vi "pulsedRead.vi"(0 "osc in":refnum<visa-resource-name>, 1 "connection ID":refnum<k5>, 2 "recCycles":u64=40, 5 "channel":u8, 6 "error in (no error)":errorcluster, 7 "freq (MHz)":dbl=1.367, 9 "cycles":u64=30, 11 "points":u64=80000, 12 "SEQ IN":u32) -> (3 "connection ID out":refnum<k5>, 4 "osc out":refnum<visa-resource-name>, 10 "error out":errorcluster, 13 "voltage":dbl[](array[numeric]), 14 "SEQ OUT":u32, 15 "time":dbl[](array[numeric]))   [LabVIEW 2016]
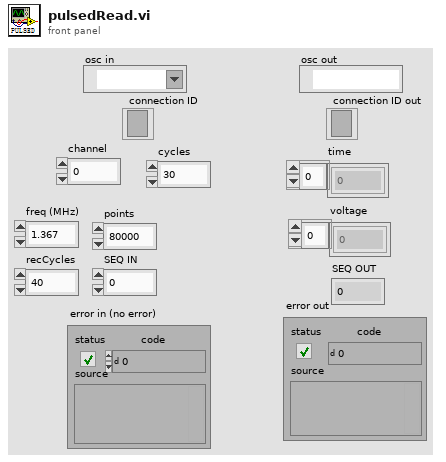
[diagram p1: front panel]
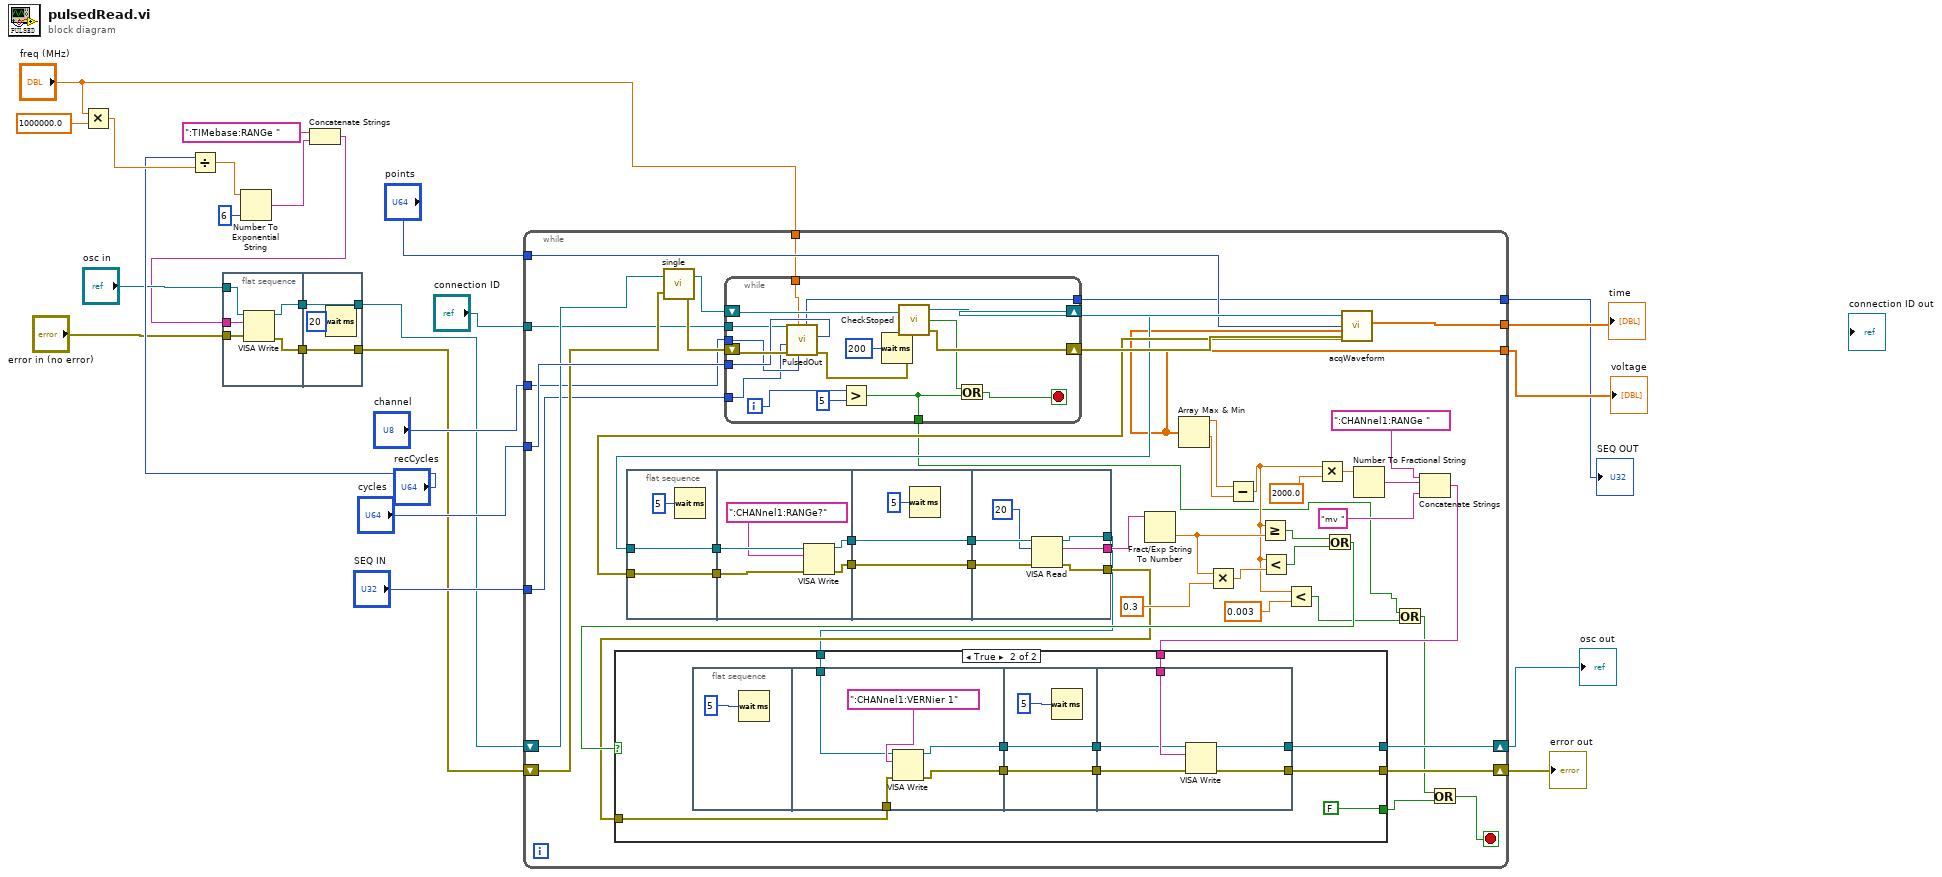
[diagram p0: block diagram]
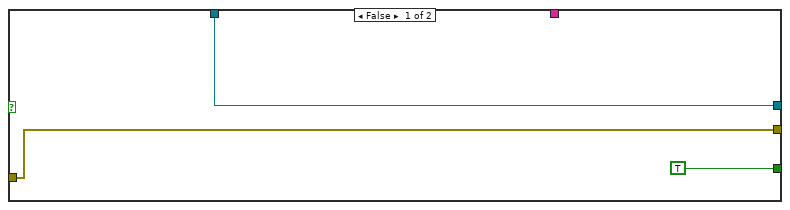
[diagram p2: hidden frame]
diagram:
  n1 = Multiply(x="freq (MHz)", y=1000000.0) -> (x*y=w13:dbl)
  n2 = Divide(x="recCycles", y=w13) -> (x/y=w11:dbl)
  n3 = flat-sequence {
    tunnel: "osc in" -> [w30]
    tunnel: w6 -> [w29]
    tunnel: "error in (no error)" -> [w28]
    tunnel: [w27] -> w4
    tunnel: [w26] -> w2
    tunnel: [w33] -> w3
    tunnel: w4 -> [w33]
    tunnel: [w32] -> w1
    tunnel: w2 -> [w32]
    frame #0 {
      n4 = VISA Write(VISA resource name=w30, write buffer=w29, error in (no error)=w28) -> (VISA resource name out=w26:refnum<visa-resource-name>, error out=w27:errorcluster)  [unwired: 1 out]
    }
    frame #1 {
      n5 = Wait (ms)(milliseconds to wait=u32 20) -> ()  [unwired: 1 out]
    }
  }
  n6 = Number To Exponential String(number=w11, precision (6)=i16 6) -> (E-format string=w8:string)  [unwired: 2 in]
  n7 = Concatenate Strings(":TIMebase:RANGe " ("string"), w8) -> (w6:string)
  n8 = while {
    tunnel: "points" -> [w74]
    tunnel: [w54] -> w22
    tunnel: [w53] -> w23
    shift-right: [w52] -> w21
    shift-left: w1 -> [w49]
    shift-right: [w51] -> w24
    shift-left: w3 -> [w47]
    tunnel: "cycles" -> [w50]
    tunnel: "channel" -> [w45]
    tunnel: "connection ID" -> [w37]
    tunnel: "SEQ IN" -> [w36]
    tunnel: [w35] -> w16
    tunnel: "freq (MHz)" -> [w34]
    stop <- w43 stop-if-true
    n9 = flat-sequence {
      tunnel: w72 -> [w111]
      tunnel: w73 -> [w112]
      tunnel: [w112] -> w82
      tunnel: [w111] -> w81
      tunnel: w82 -> [w117]
      tunnel: w81 -> [w116]
      tunnel: [w114] -> w80
      tunnel: [w113] -> w79
      tunnel: [w119] -> w78
      tunnel: w80 -> [w119]
      tunnel: [w118] -> w77
      tunnel: w79 -> [w118]
      tunnel: w78 -> [w126]
      tunnel: w77 -> [w125]
      tunnel: [w124] -> w71
      tunnel: [w123] -> w62
      tunnel: [w122] -> w61
      frame #0 {
        n10 = Wait (ms)(milliseconds to wait=u32 5) -> ()  [unwired: 1 out]
      }
      frame #1 {
        n11 = VISA Write(VISA resource name=w116, write buffer=":CHANnel1:RANGe?", error in (no error)=w117) -> (VISA resource name out=w114:refnum<visa-resource-name>, error out=w113:errorcluster)  [unwired: 1 out]
      }
      frame #2 {
        n12 = Wait (ms)(milliseconds to wait=u32 5) -> ()  [unwired: 1 out]
      }
      frame #3 {
        n13 = VISA Read(VISA resource name=w126, byte count=20, error in (no error)=w125) -> (VISA resource name out=w122:refnum<visa-resource-name>, read buffer=w124:string, error out=w123:errorcluster)  [unwired: 1 out]
      }
    }
    n14 = call "single.vi"("error in (no error)"=w47, "OSC in"=w49) -> ("error out"=w46:errorcluster, "OSC out"=w48:refnum<visa-resource-name>)
    n15 = while {
      shift-right: [w139] -> w75
      shift-left: w46 -> [w143]
      shift-right: [w140] -> w76
      shift-left: w48 -> [w142]
      tunnel: w50 -> [w137]
      tunnel: w45 -> [w136]
      tunnel: [w131] -> w40
      tunnel: w37 -> [w130]
      tunnel: w36 -> [w129]
      tunnel: [w128] -> w35
      tunnel: w34 -> [w127]
      i -> [w134]
      stop <- w132 stop-if-true
      n16 = call "PulsedOut.vi"("Cycles"=w137, "Channel"=w136, "frequency (MHz)"=w127, "error in (no error)"=w143, "SEQ IN"=w129, "connection ID"=w130) -> ("error out"=w141:errorcluster, "SEQ OUT"=w128:u32)  [unwired: 1 in, 2 out]
      n17 = Greater?(x=w134, y=5) -> (0:w131:bool)
      n18 = Wait (ms)(milliseconds to wait=u32 200) -> ()  [unwired: 1 out]
      n19 = call "CheckStoped.vi"("OSC in"=w142, "error in (no error)"=w141) -> ("OSC out"=w140:refnum<visa-resource-name>, "Stopped?"=w135:bool, "error out"=w139:errorcluster)
      n20 = Or(x=w135, y=w131) -> (x .or. y?=w132:bool)
    }
    n21 = Fract/Exp String To Number(string=w71) -> (number=w68:dbl)  [unwired: 3 in, 1 out]
    n22 = Multiply(x=w68, y=0.3) -> (x*y=w66:dbl)
    n23 = call "acqWaveform.vi"("OSC in"=w76, "Points"=w74, "error in (no error)"=w75) -> ("OSC out"=w72:refnum<visa-resource-name>, "time sequence"=w53:dbl[], "Voltage sequence"=w54:dbl[], "error out"=w73:errorcluster)
    n24 = Array Max & Min(array=w54) -> (max value=w70:dbl, min value=w69:dbl)  [unwired: 2 out]
    n25 = Subtract(x=w70, y=w69) -> (x-y=w42:dbl)
    n26 = Greater Or Equal?(x=w42, y=w68) -> (x >= y?=w65:bool)
    n27 = Less?(x=w42, y=w66) -> (x < y?=w64:bool)
    n28 = Less?(x=w42, y=0.003) -> (x < y?=w38:bool)
    n29 = Multiply(x=w42, y=2000.0) -> (x*y=w59:dbl)
    n30 = Or(x=w65, y=w64) -> (x .or. y?=w63:bool)
    n31 = Number To Fractional String(number=w59) -> (F-format string=w57:string)  [unwired: 3 in]
    n32 = Or(x=w40, y=w38) -> (x .or. y?=w39:bool)
    n33 = Concatenate Strings(":CHANnel1:RANGe ", w57, "mv ") -> (w55:string)
    n34 = case shown="True" w63 {
      tunnel: w62 -> [w84 w95]
      tunnel: w61 -> [w85 w94]
      tunnel: w55 -> [_ w93]
      tunnel: [w85 w88] -> w52
      tunnel: [w84 w87] -> w51
      tunnel: [TRUE FALSE] -> w44
      frame False {
      }
      frame True {
        n35 = flat-sequence {
          tunnel: w95 -> [w100]
          tunnel: w94 -> [w99]
          tunnel: [w98] -> w91
          tunnel: [w97] -> w89
          tunnel: [w103] -> w92
          tunnel: w91 -> [w103]
          tunnel: [w102] -> w90
          tunnel: w89 -> [w102]
          tunnel: w93 -> [w109]
          tunnel: w92 -> [w108]
          tunnel: w90 -> [w107]
          tunnel: [w106] -> w88
          tunnel: [w105] -> w87
          frame #0 {
            n36 = Wait (ms)(milliseconds to wait=u32 5) -> ()  [unwired: 1 out]
          }
          frame #1 {
            n37 = VISA Write(VISA resource name=w99, write buffer=":CHANnel1:VERNier 1", error in (no error)=w100) -> (VISA resource name out=w98:refnum<visa-resource-name>, error out=w97:errorcluster)  [unwired: 1 out]
          }
          frame #2 {
            n38 = Wait (ms)(milliseconds to wait=u32 5) -> ()  [unwired: 1 out]
          }
          frame #3 {
            n39 = VISA Write(VISA resource name=w108, write buffer=w109, error in (no error)=w107) -> (VISA resource name out=w106:refnum<visa-resource-name>, error out=w105:errorcluster)  [unwired: 1 out]
          }
        }
      }
    }
    n40 = Or(x=w39, y=w44) -> (x .or. y?=w43:bool)
  }
  "error out" <- w24
  "time" <- w23
  "osc out" <- w21
  "voltage" <- w22
  "SEQ OUT" <- w16
